vi "get shift no..vi"() -> (2 "SHIFT":string)   [LabVIEW 2015]
panel:
  out "Minutes":string
  out "Hour":string
  out "date time rec":T1
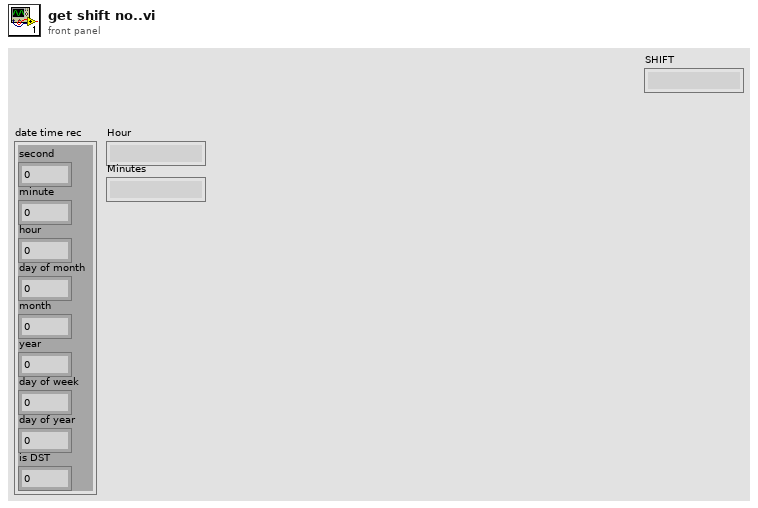
[diagram p1: front panel]
types:
  T1 = cluster{"second":i32, "minute":i32, "hour":i32, "day of month":i32, "month":i32, "year":i32, "day of week":i32, "day of year":i32, "is DST":i32}
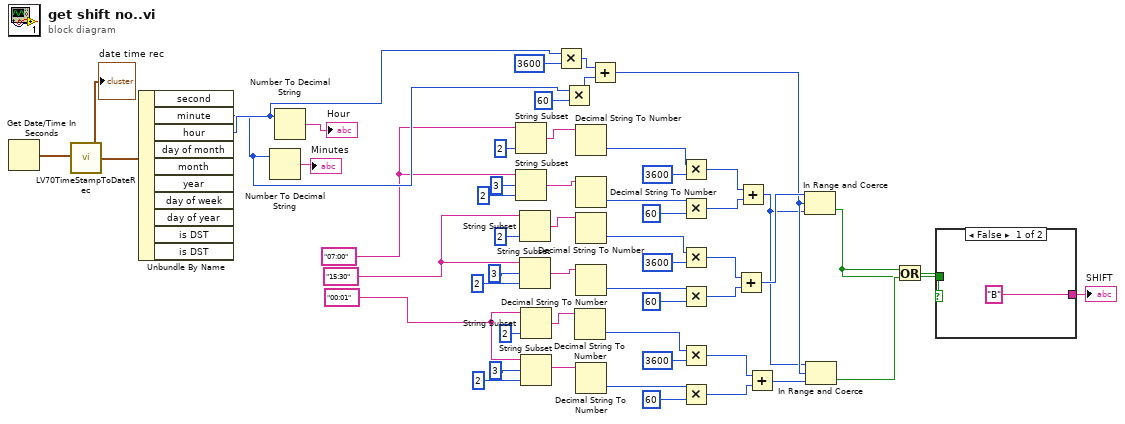
[diagram p0: block diagram]
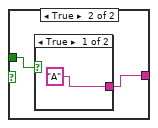
[diagram p2: hidden frame]
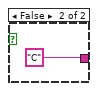
[diagram p3: hidden frame]
diagram:
  w2 = "00:01" ("SHIFT A START TIME")
  w3 = "15:30" ("SHIFT A START TIME")
  w4 = "07:00" ("SHIFT A START TIME")
  n1 = Get Date/Time In Seconds() -> (seconds since 1Jan1904=w54:timestamp)
  n2 = call <vilib>:"LV70TimeStampToDateRec.vi"("time stamp"=w54) -> ("date time rec"=w53:T1)
  "date time rec" <- w53
  n3 = Unbundle By Name(w53) -> ("minute"=w40:i32, "hour"=w41:i32)  [unwired: 8 out]
  n4 = Number To Decimal String(number=w40) -> (decimal integer string=→"Minutes":string)  [unwired: 1 out]
  n5 = Number To Decimal String(number=w41) -> (decimal integer string=→"Hour":string)  [unwired: 1 out]
  n6 = String Subset(string=w4, length (rest)=2 ("length (rest)")) -> (substring=w39:string)  [unwired: 1 out]
  n7 = String Subset(string=w4, offset (0)=3 ("length (rest)"), length (rest)=2 ("length (rest)")) -> (substring=w35:string)
  n8 = String Subset(string=w3, length (rest)=2 ("length (rest)")) -> (substring=w17:string)  [unwired: 1 out]
  n9 = String Subset(string=w3, offset (0)=3 ("length (rest)"), length (rest)=2 ("length (rest)")) -> (substring=w16:string)
  n10 = String Subset(string=w2, length (rest)=2 ("length (rest)")) -> (substring=w26:string)  [unwired: 1 out]
  n11 = String Subset(string=w2, offset (0)=3 ("length (rest)"), length (rest)=2 ("length (rest)")) -> (substring=w25:string)
  n12 = Multiply(x=w41, y=3600) -> (x*y=w8:i32)
  n13 = Multiply(x=w40, y=60) -> (x*y=w7:i32)
  n14 = Decimal String To Number(string=w26) -> (number=w27:i32)  [unwired: 3 out]
  n15 = Decimal String To Number(string=w39) -> (number=w38:i32)  [unwired: 3 out]
  n16 = Decimal String To Number(string=w35) -> (number=w34:i32)  [unwired: 3 out]
  n17 = Decimal String To Number(string=w17) -> (number=w18:i32)  [unwired: 3 out]
  n18 = Decimal String To Number(string=w16) -> (number=w21:i32)  [unwired: 3 out]
  n19 = Decimal String To Number(string=w25) -> (number=w29:i32)  [unwired: 3 out]
  n20 = Add(x=w8, y=w7) -> (x+y=w14:i32)
  n21 = Multiply(x=w38, y=3600) -> (x*y=w33:i32)
  n22 = Multiply(x=w34, y=60) -> (x*y=w32:i32)
  n23 = Multiply(x=w18, y=3600) -> (x*y=w22:i32)
  n24 = Multiply(x=w21, y=60) -> (x*y=w23:i32)
  n25 = Multiply(x=w27, y=3600) -> (x*y=w30:i32)
  n26 = Multiply(x=w29, y=60) -> (x*y=w31:i32)
  n27 = Add(x=w22, y=w23) -> (x+y=w15:i32)
  n28 = Add(x=w33, y=w32) -> (x+y=w6:i32)
  n29 = Add(x=w30, y=w31) -> (x+y=w5:i32)
  n30 = In Range and Coerce(upper limit=w15, x=w14, lower limit=w6) -> (In Range?=w12:bool)  [unwired: 1 out]
  n31 = In Range and Coerce(upper limit=w6, x=w14, lower limit=w5) -> (In Range?=w13:bool)  [unwired: 1 out]
  n32 = Or(x=w12, y=w13) -> (x .or. y?=w11:bool)
  n33 = case shown="False" w11 {
    tunnel: ["B" w57] -> w1
    tunnel: w12 -> [_ w56]
    frame False {
    }
    frame True {
      n34 = case shown="True" w56 {
        tunnel: ["A" "C"] -> w57
        frame True {
        }
        frame False {
        }
      }
    }
  }
  "SHIFT" <- w1
